vi "Actor Core.vi"(8 "error in":errorcluster, 11 "Nested in":refnum<class "Monedas.lvclass">) -> (0 "error out":errorcluster, 3 "Actor out":refnum<class "Actor.lvclass">)   [LabVIEW 2021, in "Monedas.lvlib" / "Monedas.lvclass"]
doc: "(<B>Filename</B>: Actor Framework.lvlib:Actor.lvclass:Actor Core.vi)\n\nReceives messages to the actor, reacts to them, and initiates any error handling that may shut the actor down.\n\nDescendant classes may override this VI to append parallel tasks for the actor to complete while it handles messages. Overrides use the Call Parent Method node."
uses:
  Monedas.lvclass
  C:/Program Files (x86)/National Instruments/LabVIEW 2021/vi.lib/ActorFramework/Actor/Actor.lvclass
  <vilib>/ActorFramework/Actor/Actor.lvclass
  <vilib>/ActorFramework/Actor/Actor.lvclass/Actor.ctl
  <vilib>/ActorFramework/Message Enqueuer/Message Enqueuer.lvclass/Message Enqueuer.ctl
  Monedas.lvclass/Monedas.ctl
  Monedas Messages/Credito de Monedas Msg/Credito de Monedas Msg.lvclass/Credito de Monedas Msg.ctl
  <vilib>/ActorFramework/Message Enqueuer/Init from Existing Queue.vi
  <vilib>/ActorFramework/Message Enqueuer/Enqueue.vi
  <vilib>/ActorFramework/Stop Msg/Stop Msg.lvclass
  C:/Program Files (x86)/National Instruments/LabVIEW 2021/vi.lib/ActorFramework/Message/Message.lvclass
  Monedas Messages/Credito de Monedas Msg/Credito de Monedas Msg.lvclass
  <vilib>/ActorFramework/Message Priority Queue/Priority Enqueue.vi
  <vilib>/ActorFramework/Message Enqueuer/Message Enqueuer.lvclass
  C:/Users/scrap/Fork/Vending Machine AF/Actor-Framework-Vending-Machine/Vending Machine AF Folder/Monedas/Monedas.lvclass
panel:
  out "Credito total":string
  in  "10 pesos":bool
  in  "5 pesos":bool
  in  "2 pesos":bool
  in  "1 peso":bool
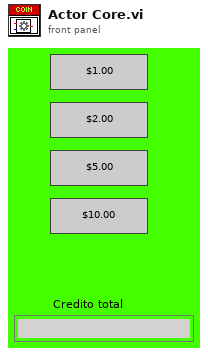
[diagram p1: front panel]
types:
  T1 = cluster{"Stop":refnum<user-event>, "Credito total":refnum<user-event>}
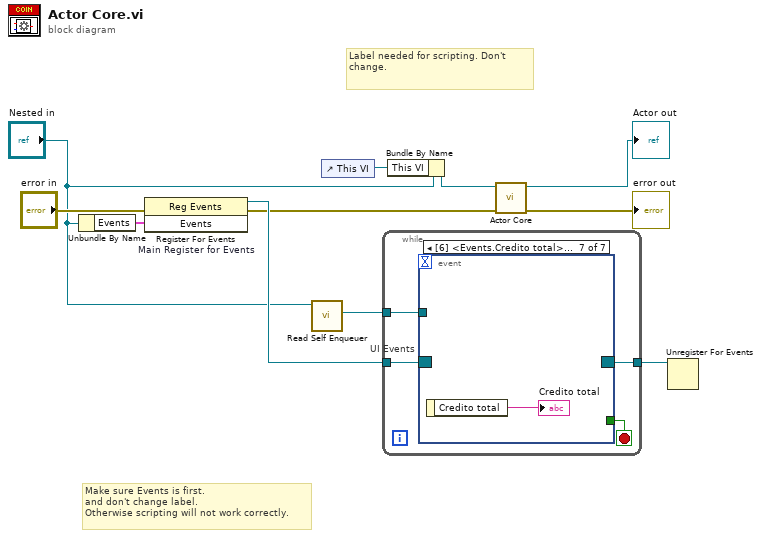
[diagram p0: block diagram]
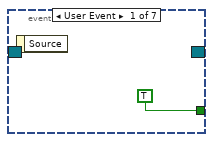
[diagram p2: hidden frame]
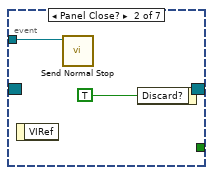
[diagram p3: hidden frame]
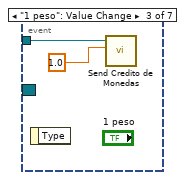
[diagram p4: hidden frame]
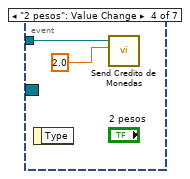
[diagram p5: hidden frame]
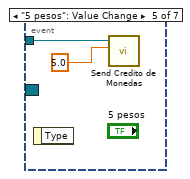
[diagram p6: hidden frame]
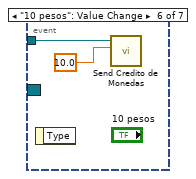
[diagram p7: hidden frame]
diagram:
  # "Label needed for scripting. Don't change."
  # "Make sure Events is first.\nand don't change label.\nOtherwise scripting will not work correctly."
  n1 = Unbundle By Name("Nested in") -> ("Events"=w8:T1)
  n2 = register-events "Main Register for Events"(error in="error in", w8) -> (reference out=w9:refnum<event-registration>, error out=w4:errorcluster)  [unwired: 1 in]
  n3 = call <vilib>:"Read Self Enqueuer.vi"("Actor"="Nested in") -> ("Self Enqueuer"=w6:refnum<class "Message Enqueuer.lvclass">)  [unwired: 10 in]
  n4 = control-ref of="This VI"() -> (w2:refnum<vi>)
  n5 = while {
    tunnel: w9 -> [w15]
    tunnel: [w13] -> w7
    tunnel: w6 -> [w12]
    stop <- w14 stop-if-true
    n6 = event "UI Events" shown="[6] <Events.Credito total>: User Event" {
      selector: w15 -> [_ _ _ _ _ _ _]
      dyn-events: [_ _ _ _ _ _ _] -> w13
      timeout: _ -> [_ _ _ _ _ _ _]
      tunnel: [TRUE _ _ _ _ _ _] -> w14
      tunnel: w12 -> [_ w17 w20 w22 w24 w26 _]
      event User Event {
        n7 = event-data() -> ()  [unwired: 1 in, 1 out]
      }
      event Panel Close? {
        n8 = event-data() -> ()  [unwired: 1 in, 1 out]
        n9 = call <vilib>:"Send Normal Stop.vi"("Message Enqueuer"=w17) -> ()  [unwired: 10 in, 1 out]
        n10 = event-data("Discard?"=TRUE) -> ()  [unwired: 1 in, 1 out]
      }
      event "1 peso": Value Change {
        n11 = event-data() -> ()  [unwired: 1 in, 1 out]
        n12 = call "Send Credito de Monedas.vi"("Dinero"=1.0, "Message Enqueuer"=w20) -> ()  [unwired: 8 in, 2 out]
      }
      event "2 pesos": Value Change {
        n13 = event-data() -> ()  [unwired: 1 in, 1 out]
        n14 = call "Send Credito de Monedas.vi"("Dinero"=2.0, "Message Enqueuer"=w22) -> ()  [unwired: 8 in, 2 out]
      }
      event "5 pesos": Value Change {
        n15 = event-data() -> ()  [unwired: 1 in, 1 out]
        n16 = call "Send Credito de Monedas.vi"("Dinero"=5.0, "Message Enqueuer"=w24) -> ()  [unwired: 8 in, 2 out]
      }
      event "10 pesos": Value Change {
        n17 = event-data() -> ()  [unwired: 1 in, 1 out]
        n18 = call "Send Credito de Monedas.vi"("Dinero"=10.0, "Message Enqueuer"=w26) -> ()  [unwired: 8 in, 2 out]
      }
      event User Event {
        n19 = event-data() -> ("Credito total"=→"Credito total":string)  [unwired: 1 in]
      }
    }
  }
  n20 = Bundle By Name(cluster="Nested in", "This VI"=w2) -> (w3:refnum<class "Monedas.lvclass">)
  n21 = call-parent "Actor Core.vi"("error in"=w4, "Actor in"=w3) -> ("error out"=→"error out":errorcluster, "Actor out"=→"Actor out":refnum<class "Actor.lvclass">)  [unwired: 8 in]
  n22 = Unregister For Events(event registration refnum=w7) -> ()  [unwired: 1 in, 1 out]
